vi "TCP Port Monitor.vi"() -> ()   [LabVIEW 2020]
uses:
  <vilib>/regexp/Match Regular Expression.xnode
panel:
  out "Graph":dbl[][](graph)
  in  "stop":bool
  out "Array":T1(array[cluster])
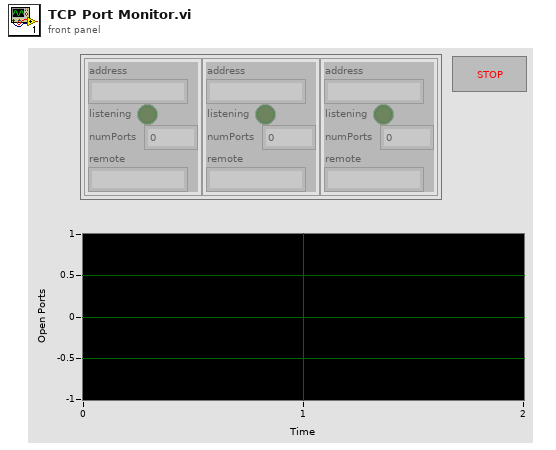
[diagram p1: front panel]
types:
  T1 = cluster{"address":string, "listening":bool, "numPorts":i32, "remote":string}[]
  T2 = cluster{"address":string, "listening":bool, "numPorts":i32, "remote":string}
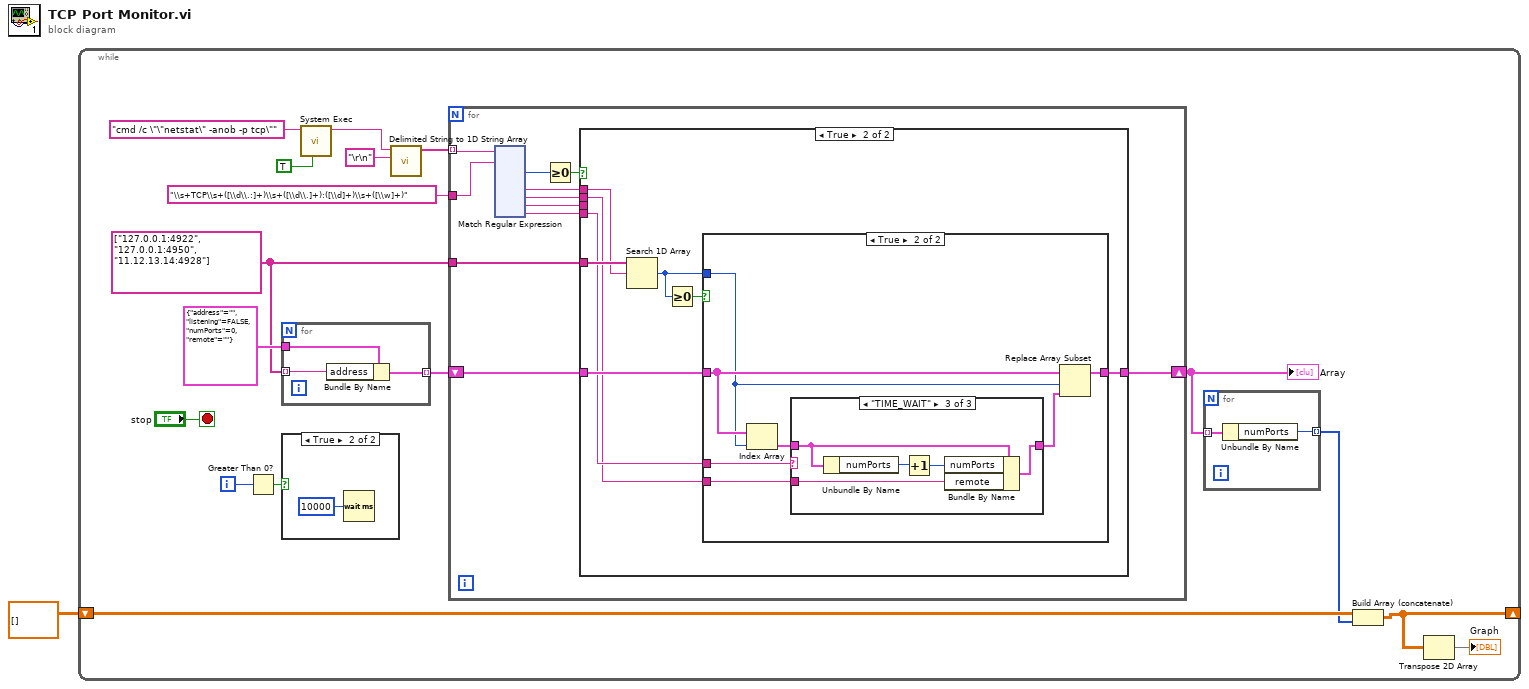
[diagram p0: block diagram]
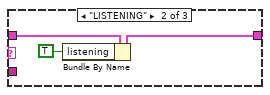
[diagram p6: hidden frame]
diagram:
  n1 = while {
    shift-right: [w3] -> _
    shift-left: dbl[][] [] ("Waveform Graph") -> [w5]
    i -> [w9]
    stop <- "stop" stop-if-true
    w7 = string[] ["127.0.0.1:4922", "127.0.0.1:4950", "11.12.13.14:4928"]
    n2 = Greater Than 0?(x=w9) -> (x > 0?=w8:bool)
    n3 = for {
      tunnel: w7 -> [w23] mode=indexing
      tunnel: T2 {"address"="", "listening"=FALSE, "numPorts"=0, "remote"=""} -> [w24]
      tunnel: [w22] -> w11 mode=indexing
      n4 = Bundle By Name(cluster=w24, "address"=w23) -> (w22:T2)
    }
    n5 = case shown="True" w8 {
      frame False {
      }
      frame True {
        n6 = Wait (ms)(milliseconds to wait=u32 10000) -> ()  [unwired: 1 out]
      }
    }
    n7 = call <vilib>:"System Exec.vi"("run minimized? (F)"=TRUE, "command line"="cmd /c \"\"netstat\" -anob -p tcp\"") -> ("standard output"=w16:string)  [unwired: 6 in, 3 out]
    n8 = call <vilib>:"Delimited String to 1D String Array.vi"("delimiter"="\r\n" ("search string/char (-)"), "delimited string"=w16) -> ("string array"=w14:string[])  [unwired: 9 in]
    n9 = for {
      tunnel: w14 -> [w35] mode=indexing
      tunnel: "\\s+TCP\\s+([\\d\\.:]+)\\s+([\\d\\.]+):([\\d]+)\\s+([\\w]+)" ("regular expression") -> [w34]
      tunnel: w7 -> [w27]
      shift-right: [w25] -> w6
      shift-left: w11 -> [w26]
      n10 = xnode "Match Regular Expression"("input string"=w35, "regular expression"=w34) -> ("offset past match"=w33:i32, "submatch 1"=w32:string, "submatch 2"=w30:string, "submatch 3"=w29:string, "submatch 4"=w28:string)  [unwired: 4 in, 4 out]
      n11 = Greater Or Equal To 0?(x=w33) -> (x >= 0?=w31:bool)
      n12 = case shown="True" w31 {
        tunnel: w32 -> [_ w43]
        tunnel: w30 -> [_ w37]
        tunnel: w29 -> [_ _]
        tunnel: w28 -> [_ w39]
        tunnel: w27 -> [_ w44]
        tunnel: w26 -> [w36 w40]
        tunnel: [w36 w38] -> w25
        frame False {
        }
        frame True {
          n13 = Search 1D Array(1D array=w44, element=w43) -> (index of element=w41:i32)  [unwired: 1 in]
          n14 = Greater Or Equal To 0?(x=w41) -> (x >= 0?=w42:bool)
          n15 = case shown="True" w42 {
            tunnel: w41 -> [_ w48]
            tunnel: w40 -> [w45 w50]
            tunnel: w39 -> [_ w52]
            tunnel: [w45 w47] -> w38
            tunnel: w37 -> [_ w46]
            frame False {
            }
            frame True {
              n16 = Index Array(array=w50, index=w48) -> (element=w51:T2)
              n17 = case shown="\"TIME_WAIT\"" w52 {
                tunnel: w51 -> [w53 w56 w60]
                tunnel: [w53 w54 w61] -> w49
                tunnel: w46 -> [_ _ w57]
                frame "", Default {
                }
                frame "LISTENING" {
                  n18 = Bundle By Name(cluster=w56, "listening"=TRUE) -> (w54:T2)
                }
                frame "TIME_WAIT" {
                  n19 = Unbundle By Name(w60) -> ("numPorts"=w59:i32)
                  n20 = Increment(x=w59) -> (x+1=w58:i32)
                  n21 = Bundle By Name(cluster=w60, "numPorts"=w58, "remote"=w57) -> (w61:T2)
                }
              }
              n22 = Replace Array Subset(array=w50, new element=w49, index=w48) -> (w47:T1)
            }
          }
        }
      }
    }
    "Array" <- w6
    n23 = for {
      tunnel: w6 -> [w20] mode=indexing
      tunnel: [w19] -> w4 mode=indexing
      n24 = Unbundle By Name(w20) -> ("numPorts"=w19:i32)
    }
    n25 = Build Array (concatenate)(w5, w4) -> (w3:dbl[][])
    n26 = Transpose 2D Array(2D array=w3) -> (transposed array=→"Graph":dbl[][])
  }
